vi "compressFiles.vi"(0 "show_bool_legal":bool=TRUE, 1 "original Path":path=path "S:/PNA_Data/L7KQF001-SD-R/SN-152440002_150901", 2 "重测原因":string, 3 "NetPathCompress2":path, 4 "EEPROMTF":bool=TRUE, 5 "Excel?":bool=TRUE, 6 "测试模式":string, 7 "db_VNA":string="L7KQF003-SD-R1;l7kqf003-sd-r1510090002;", 8 "P/N:":string, 9 "S/N:":string="152860001", 10 "测试线别":string, 12 "NetPathCompress1":path, 13 "NetCmdCompress":string, 14 "mis原始sn字符串":string, 15 "条码输出":string, 16 "eprm_datecode":string, 17 "eprm_dateAndsn":string, 20 "itsn_really":string, 21 "label_date":string, 23 "decimel_sn":string, 24 "label_sn":string, 25 "decimel_date":string, 27 "MO":string) -> ()   [LabVIEW 2011]
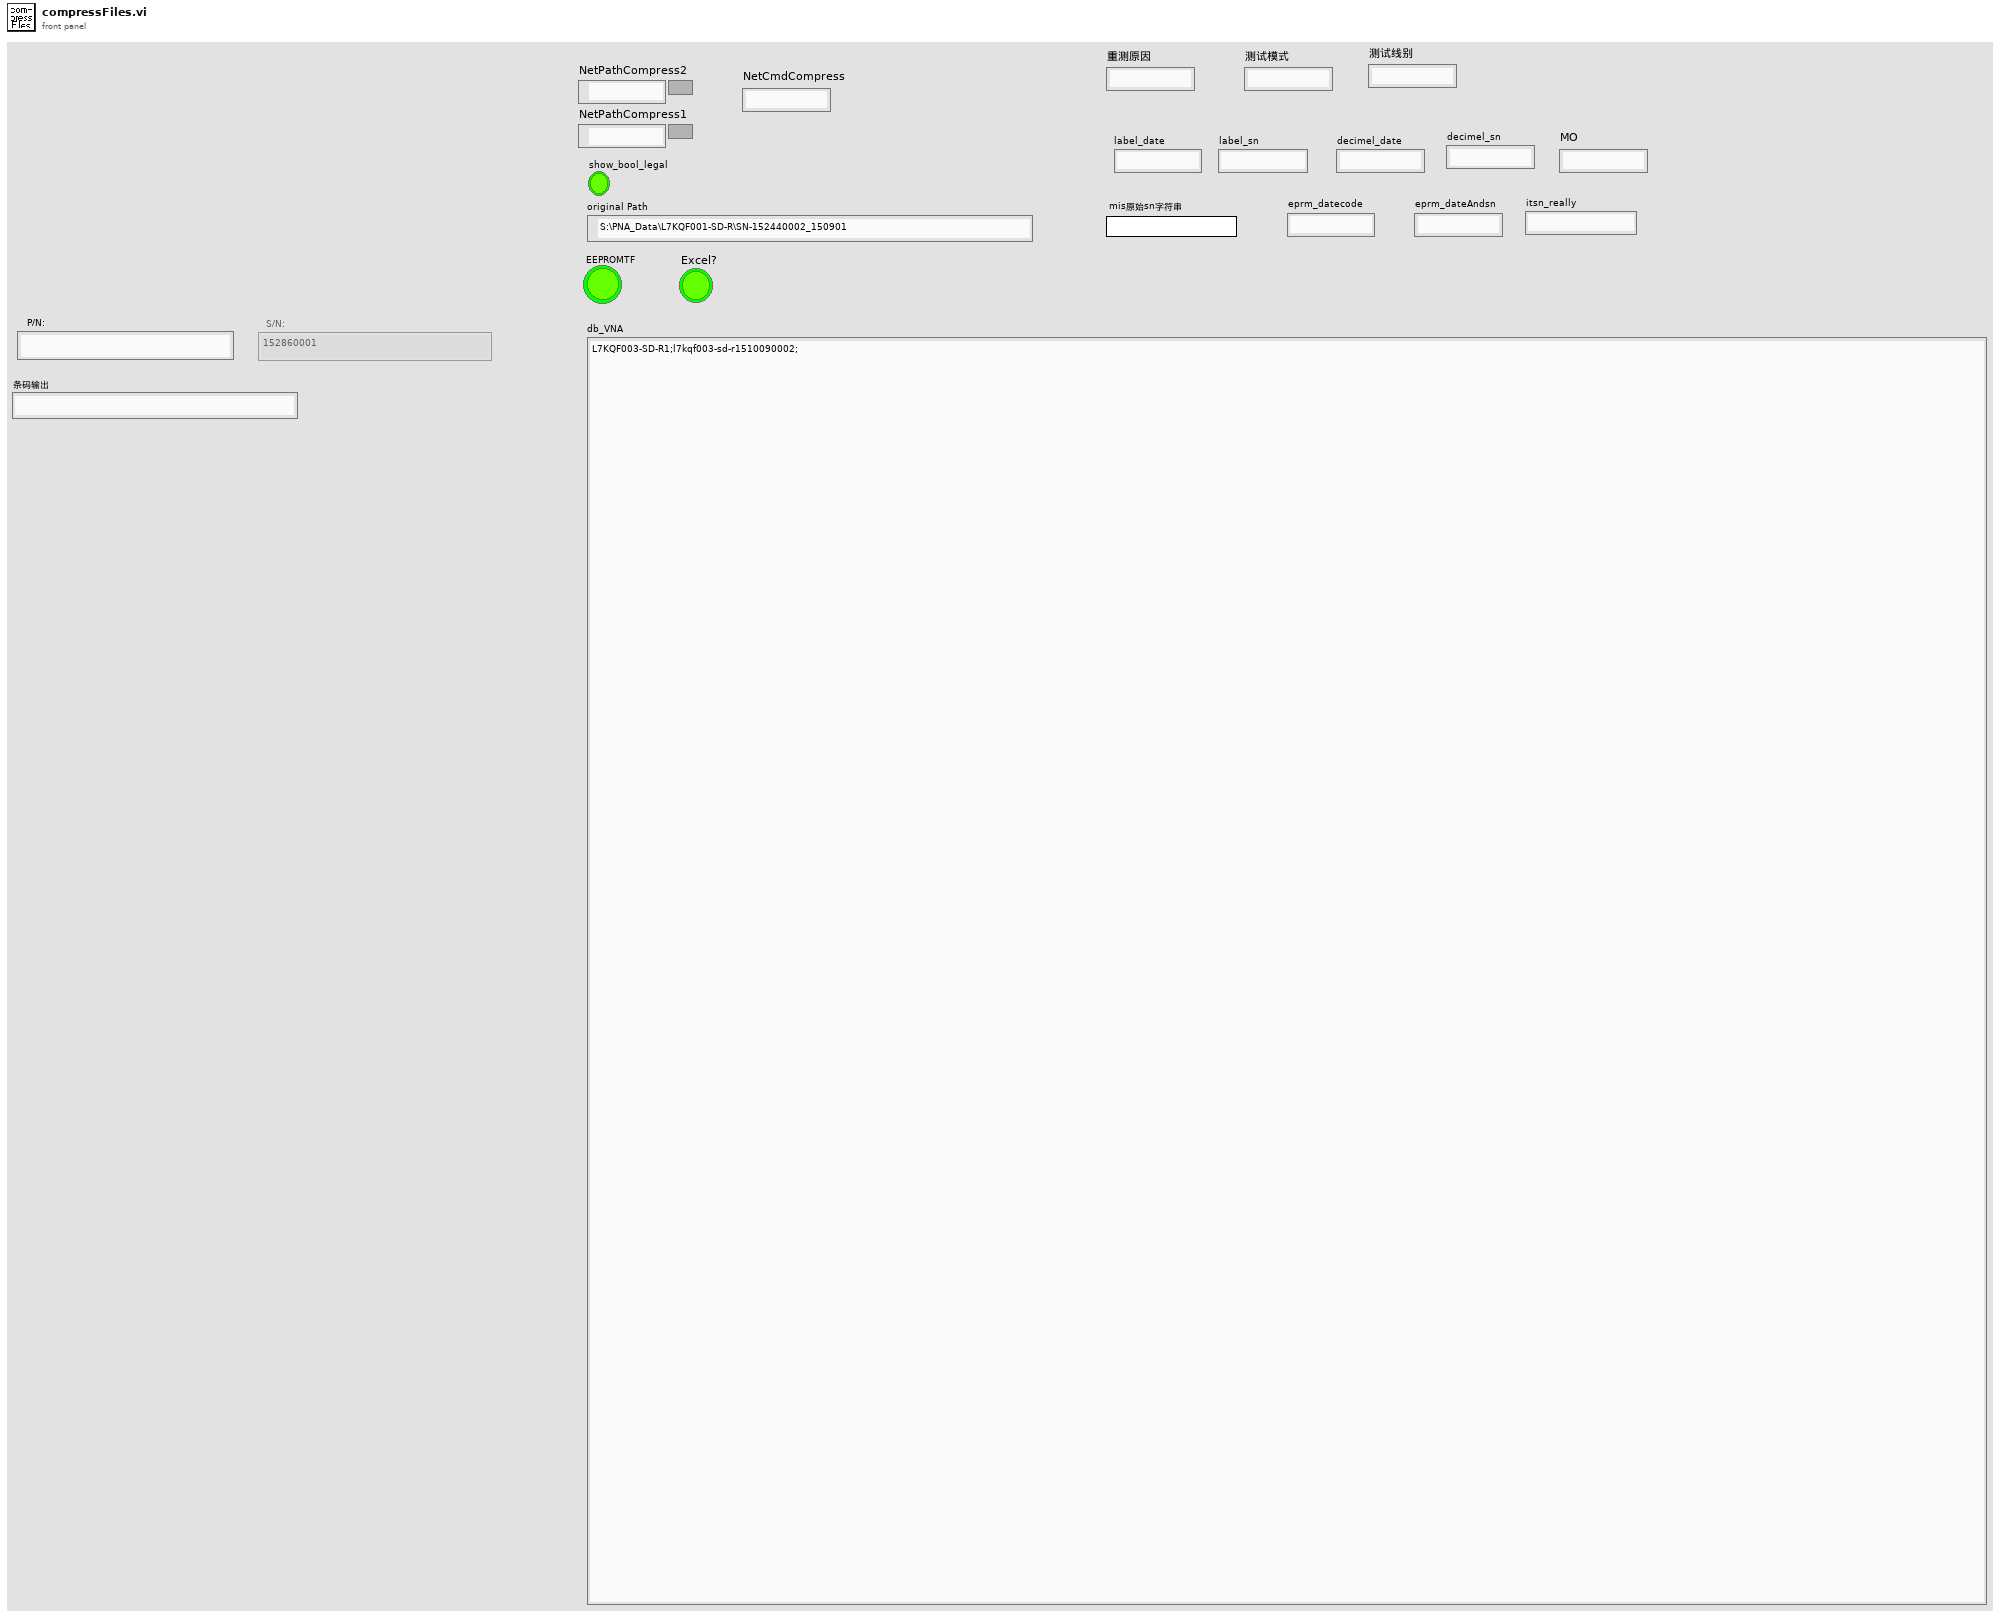
[diagram p1: front panel]
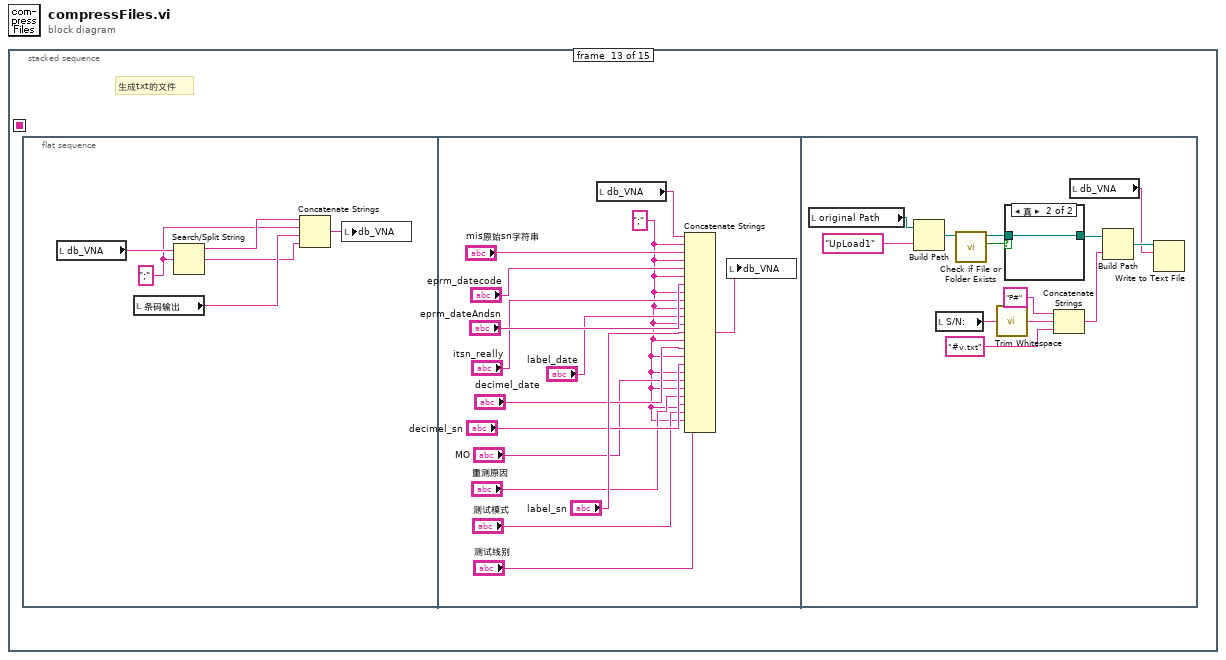
[diagram p0: block diagram]
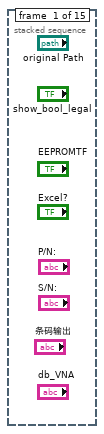
[diagram p2: hidden frame]
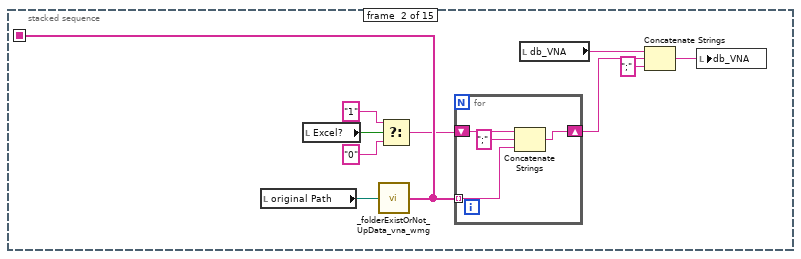
[diagram p3: hidden frame]
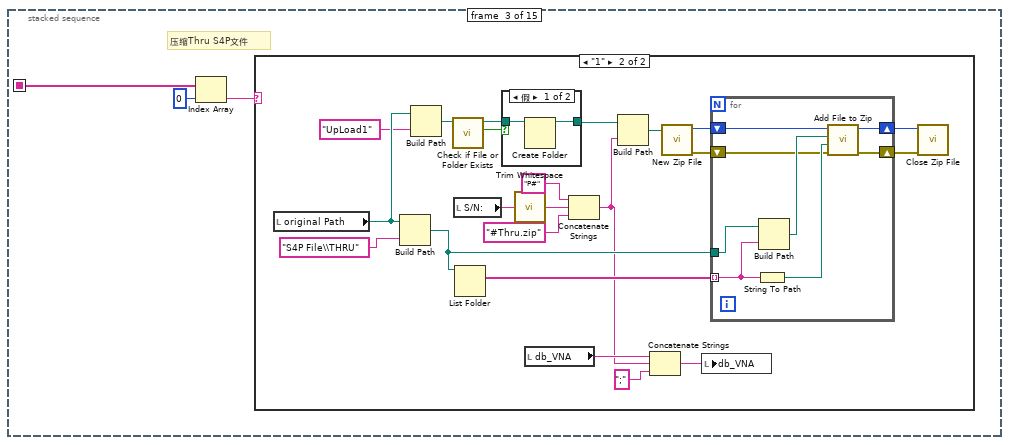
[diagram p4: hidden frame]
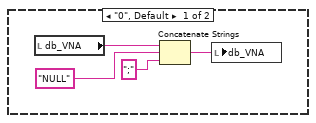
[diagram p5: hidden frame]
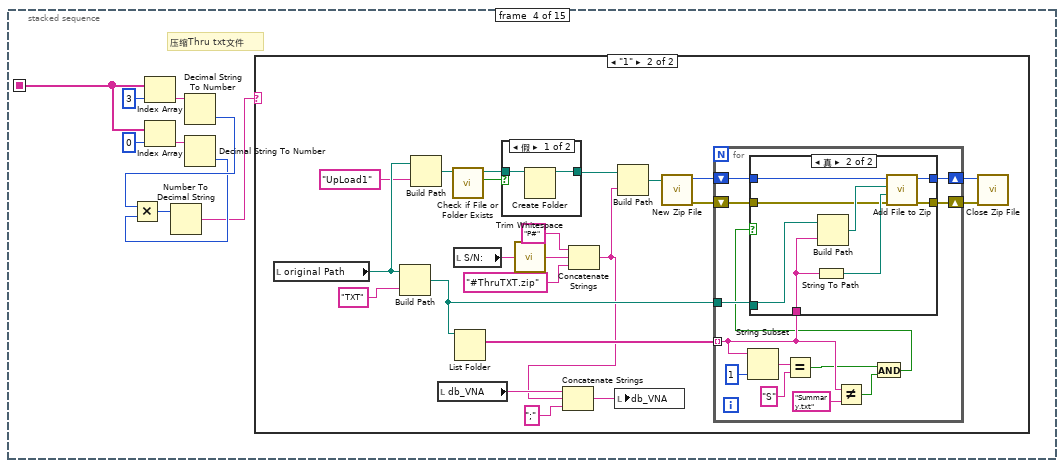
[diagram p7: hidden frame]
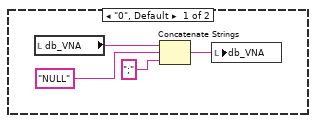
[diagram p8: hidden frame]
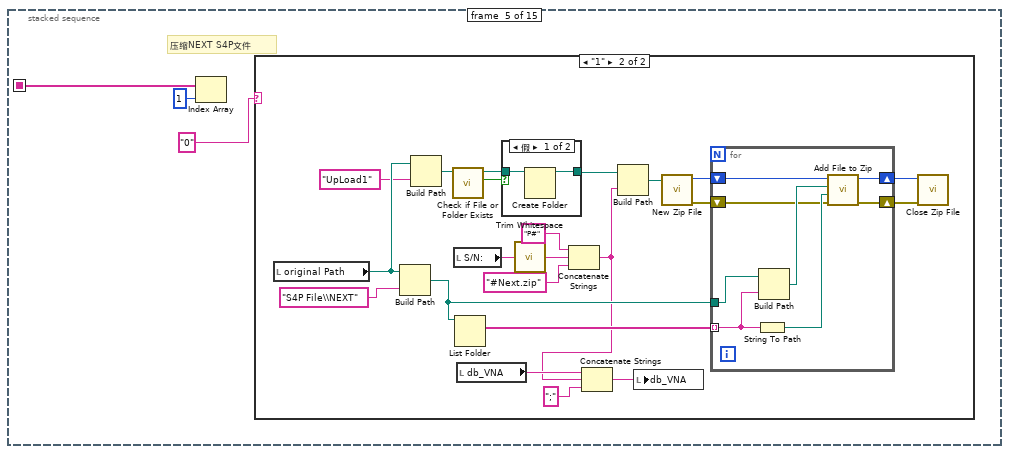
[diagram p11: hidden frame]
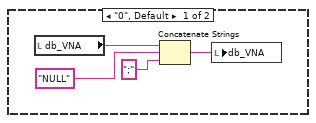
[diagram p12: hidden frame]
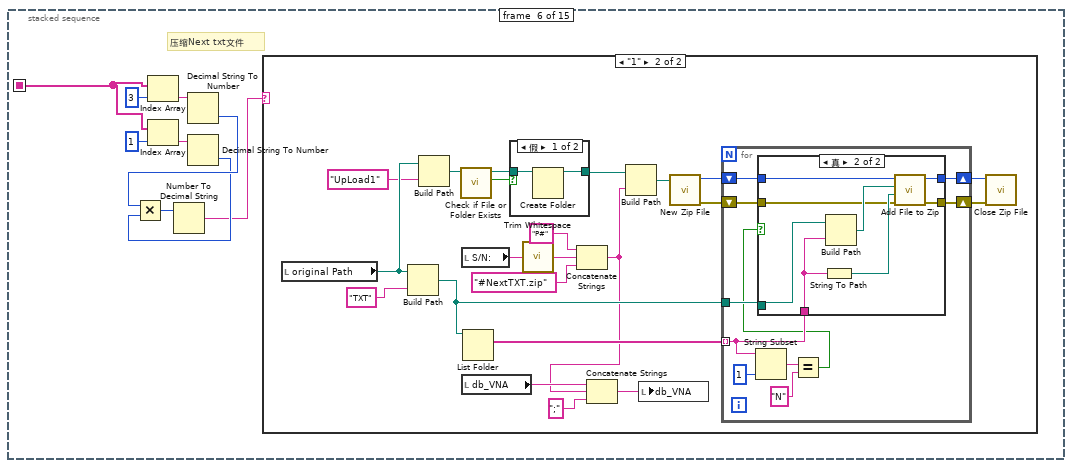
[diagram p14: hidden frame]
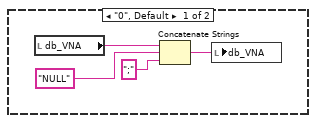
[diagram p15: hidden frame]
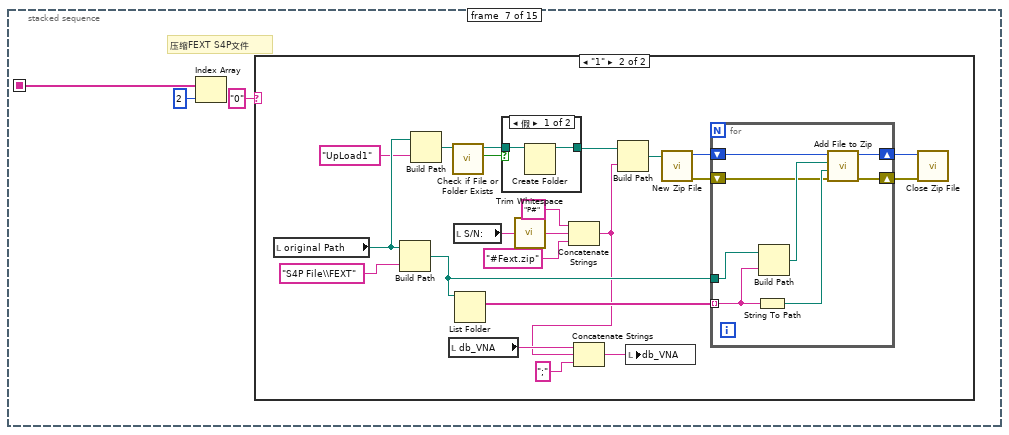
[diagram p18: hidden frame]
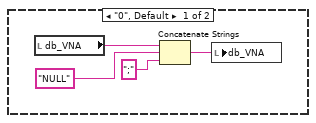
[diagram p19: hidden frame]
diagram:
  n1 = stacked-sequence {
    seq-local: [_ w2 _ _ _ _ _ _ _ _ _ _ _ _ _] -> [_ _ w17 w61 w118 w157 w216 w255 w314 w354 _ w458 _ _ _]
    frame #0 {
    }
    frame #1 {
      n2 = local read "original Path"() -> (w3:path)
      n3 = local read "Excel?"() -> (w10:bool)
      n4 = call "_folderExistOrNot_UpData_vna_wmg.vi"("基础路径"=w3) -> ("output"=w2:string[])
      n5 = Select(t="1", s=w10, f="0") -> (s? t:f=w1:string)
      n6 = for {
        tunnel: w2 -> [w12] mode=indexing
        shift-right: [w11] -> w5
        shift-left: w1 -> [w14]
        n7 = Concatenate Strings(w14, ";" ("字符串"), w12) -> (w11:string)
      }
      n8 = local read "db_VNA"() -> (w7:string)
      n9 = Concatenate Strings(w7, w5, ";" ("字符串")) -> (w6:string)
      n10 = local write "db_VNA"(w6) -> ()
    }
    frame #2 {
      # "压缩Thru S4P文件"
      n11 = Index Array(array=w17, index=0 ("索引")) -> (element=w15:string)
      n12 = case shown="\"1\"" w15 {
        frame "0", Default {
          n13 = local read "db_VNA"() -> (w21:string)
          n14 = Concatenate Strings(w21, "NULL", ";" ("字符串")) -> (w20:string)
          n15 = local write "db_VNA"(w20) -> ()
        }
        frame "1" {
          n16 = local read "original Path"() -> (w42:path)
          n17 = Build Path(base path=w42, name or relative path="S4P File\\THRU") -> (appended path=w31:path)
          n18 = Build Path(base path=w42, name or relative path="UpLoad1" ("名称或相对路径")) -> (appended path=w40:path)
          n19 = call <vilib>:"Check if File or Folder Exists.vi"("path"=w40) -> ("file or folder exists?"=w39:bool, "dup path"=w38:path)  [unwired: 8 in, 1 out]
          n20 = local read "S/N:"() -> (w37:string)
          n21 = List Folder(path=w31) -> (filenames=w32:string[])  [unwired: 3 in, 3 out]
          n22 = case shown="假" w39 {
            tunnel: w38 -> [w53 w54]
            tunnel: [w52 w54] -> w33
            frame False {
              n23 = Create Folder(path (use dialog)=w53) -> (created path=w52:path)  [unwired: 2 in, 2 out]
            }
            frame True {
            }
          }
          n24 = call <vilib>:"Trim Whitespace.vi"("string"=w37) -> ("trimmed string"=w36:string)  [unwired: 1 in]
          n25 = local read "db_VNA"() -> (w25:string)
          n26 = Concatenate Strings("P#", w36, "#Thru.zip") -> (w22:string)
          n27 = Build Path(base path=w33, name or relative path=w22) -> (appended path=w30:path)
          n28 = Concatenate Strings(w25, w22, ";" ("字符串")) -> (w24:string)
          n29 = call <vilib>:"New Zip File.vi"("target"=w30) -> ("error out"=w27:errorcluster, "zip file out"=w29:i64)  [unwired: 4 in, 1 out]
          n30 = local write "db_VNA"(w24) -> ()
          n31 = for {
            tunnel: w32 -> [w50] mode=indexing
            tunnel: w31 -> [w51]
            shift-right: [w48] -> w28
            shift-left: w29 -> [w49]
            shift-right: [w44] -> w26
            shift-left: w27 -> [w45]
            n32 = String To Path(string=w50) -> (path=w46:path)
            n33 = Build Path(base path=w51, name or relative path=w50) -> (appended path=w47:path)
            n34 = call <vilib>:"Add File to Zip.vi"("error in (no error)"=w45, "destination path in zip"=w46, "source file path"=w47, "zip file in"=w49) -> ("error out"=w44:errorcluster, "zip file out"=w48:i64)  [unwired: 6 in]
          }
          n35 = call <vilib>:"Close Zip File.vi"("error in (no error)"=w26, "zip file in"=w28) -> ()  [unwired: 5 in, 1 out]
        }
      }
    }
    frame #3 {
      # "压缩Thru txt文件"
      n36 = Index Array(array=w61, index=3 ("索引")) -> (element=w60:string)
      n37 = Index Array(array=w61, index=0 ("索引")) -> (element=w59:string)
      n38 = Decimal String To Number(string=w60) -> (number=w58:i32)  [unwired: 2 in, 1 out]
      n39 = Decimal String To Number(string=w59) -> (number=w57:i32)  [unwired: 2 in, 1 out]
      n40 = Multiply(x=w58, y=w57) -> (x*y=w56:i32)
      n41 = Number To Decimal String(number=w56) -> (decimal integer string=w55:string)  [unwired: 1 in]
      n42 = case shown="\"1\"" w55 {
        frame "0", Default {
          n43 = local read "db_VNA"() -> (w67:string)
          n44 = Concatenate Strings(w67, "NULL", ";" ("字符串")) -> (w66:string)
          n45 = local write "db_VNA"(w66) -> ()
        }
        frame "1" {
          n46 = local read "original Path"() -> (w88:path)
          n47 = Build Path(base path=w88, name or relative path="TXT") -> (appended path=w77:path)
          n48 = Build Path(base path=w88, name or relative path="UpLoad1" ("名称或相对路径")) -> (appended path=w86:path)
          n49 = local read "db_VNA"() -> (w71:string)
          n50 = call <vilib>:"Check if File or Folder Exists.vi"("path"=w86) -> ("file or folder exists?"=w85:bool, "dup path"=w84:path)  [unwired: 8 in, 1 out]
          n51 = local read "S/N:"() -> (w83:string)
          n52 = List Folder(path=w77) -> (filenames=w78:string[])  [unwired: 3 in, 3 out]
          n53 = case shown="假" w85 {
            tunnel: w84 -> [w114 w115]
            tunnel: [w113 w115] -> w79
            frame False {
              n54 = Create Folder(path (use dialog)=w114) -> (created path=w113:path)  [unwired: 2 in, 2 out]
            }
            frame True {
            }
          }
          n55 = call <vilib>:"Trim Whitespace.vi"("string"=w83) -> ("trimmed string"=w82:string)  [unwired: 1 in]
          n56 = Concatenate Strings("P#", w82, "#ThruTXT.zip") -> (w68:string)
          n57 = Concatenate Strings(w71, w68, ";" ("字符串")) -> (w70:string)
          n58 = local write "db_VNA"(w70) -> ()
          n59 = Build Path(base path=w79, name or relative path=w68) -> (appended path=w76:path)
          n60 = call <vilib>:"New Zip File.vi"("target"=w76) -> ("error out"=w73:errorcluster, "zip file out"=w75:i64)  [unwired: 4 in, 1 out]
          n61 = for {
            tunnel: w78 -> [w94] mode=indexing
            tunnel: w77 -> [w102]
            shift-right: [w100] -> w74
            shift-left: w75 -> [w101]
            shift-right: [w98] -> w72
            shift-left: w73 -> [w99]
            n62 = String Subset(string=w94, length (rest)=1 ("长度（剩余）")) -> (substring=w96:string)  [unwired: 1 in]
            n63 = Equal?(x=w96, y="S") -> (x = y?=w91:bool)
            n64 = Not Equal?(x=w94, y="Summary.txt") -> (x != y?=w92:bool)
            n65 = And(x=w91, y=w92) -> (x .and. y?=w90:bool)
            n66 = case shown="真" w90 {
              tunnel: w102 -> [_ w112]
              tunnel: w101 -> [w104 w111]
              tunnel: [w104 w110] -> w100
              tunnel: w99 -> [w103 w107]
              tunnel: [w103 w106] -> w98
              tunnel: w94 -> [_ w105]
              frame False {
              }
              frame True {
                n67 = String To Path(string=w105) -> (path=w108:path)
                n68 = Build Path(base path=w112, name or relative path=w105) -> (appended path=w109:path)
                n69 = call <vilib>:"Add File to Zip.vi"("error in (no error)"=w107, "destination path in zip"=w108, "source file path"=w109, "zip file in"=w111) -> ("error out"=w106:errorcluster, "zip file out"=w110:i64)  [unwired: 6 in]
              }
            }
          }
          n70 = call <vilib>:"Close Zip File.vi"("error in (no error)"=w72, "zip file in"=w74) -> ()  [unwired: 5 in, 1 out]
        }
      }
    }
    frame #4 {
      # "压缩NEXT S4P文件"
      n71 = Index Array(array=w118, index=1 ("索引")) -> ()  [unwired: 1 out]
      n72 = case shown="\"1\"" "0" {
        frame "0", Default {
          n73 = local read "db_VNA"() -> (w122:string)
          n74 = Concatenate Strings(w122, "NULL", ";" ("字符串")) -> (w121:string)
          n75 = local write "db_VNA"(w121) -> ()
        }
        frame "1" {
          n76 = local read "original Path"() -> (w143:path)
          n77 = Build Path(base path=w143, name or relative path="S4P File\\NEXT") -> (appended path=w132:path)
          n78 = Build Path(base path=w143, name or relative path="UpLoad1" ("名称或相对路径")) -> (appended path=w141:path)
          n79 = call <vilib>:"Check if File or Folder Exists.vi"("path"=w141) -> ("file or folder exists?"=w140:bool, "dup path"=w139:path)  [unwired: 8 in, 1 out]
          n80 = local read "S/N:"() -> (w138:string)
          n81 = List Folder(path=w132) -> (filenames=w133:string[])  [unwired: 3 in, 3 out]
          n82 = local read "db_VNA"() -> (w124:string)
          n83 = case shown="假" w140 {
            tunnel: w139 -> [w154 w155]
            tunnel: [w153 w155] -> w134
            frame False {
              n84 = Create Folder(path (use dialog)=w154) -> (created path=w153:path)  [unwired: 2 in, 2 out]
            }
            frame True {
            }
          }
          n85 = call <vilib>:"Trim Whitespace.vi"("string"=w138) -> ("trimmed string"=w137:string)  [unwired: 1 in]
          n86 = Concatenate Strings("P#", w137, "#Next.zip") -> (w123:string)
          n87 = Concatenate Strings(w124, w123, ";" ("字符串")) -> (w125:string)
          n88 = Build Path(base path=w134, name or relative path=w123) -> (appended path=w131:path)
          n89 = local write "db_VNA"(w125) -> ()
          n90 = call <vilib>:"New Zip File.vi"("target"=w131) -> ("error out"=w128:errorcluster, "zip file out"=w130:i64)  [unwired: 4 in, 1 out]
          n91 = for {
            tunnel: w133 -> [w151] mode=indexing
            tunnel: w132 -> [w152]
            shift-right: [w149] -> w129
            shift-left: w130 -> [w150]
            shift-right: [w145] -> w127
            shift-left: w128 -> [w146]
            n92 = String To Path(string=w151) -> (path=w147:path)
            n93 = Build Path(base path=w152, name or relative path=w151) -> (appended path=w148:path)
            n94 = call <vilib>:"Add File to Zip.vi"("error in (no error)"=w146, "destination path in zip"=w147, "source file path"=w148, "zip file in"=w150) -> ("error out"=w145:errorcluster, "zip file out"=w149:i64)  [unwired: 6 in]
          }
          n95 = call <vilib>:"Close Zip File.vi"("error in (no error)"=w127, "zip file in"=w129) -> ()  [unwired: 5 in, 1 out]
        }
      }
    }
    frame #5 {
      # "压缩Next txt文件"
      n96 = Index Array(array=w157, index=3 ("索引")) -> (element=w162:string)
      n97 = Index Array(array=w157, index=1 ("索引")) -> (element=w161:string)
      n98 = Decimal String To Number(string=w162) -> (number=w160:i32)  [unwired: 2 in, 1 out]
      n99 = Decimal String To Number(string=w161) -> (number=w159:i32)  [unwired: 2 in, 1 out]
      n100 = Multiply(x=w160, y=w159) -> (x*y=w158:i32)
      n101 = Number To Decimal String(number=w158) -> (decimal integer string=w156:string)  [unwired: 1 in]
      n102 = case shown="\"1\"" w156 {
        frame "0", Default {
          n103 = local read "db_VNA"() -> (w168:string)
          n104 = Concatenate Strings(w168, "NULL", ";" ("字符串")) -> (w167:string)
          n105 = local write "db_VNA"(w167) -> ()
        }
        frame "1" {
          n106 = local read "original Path"() -> (w189:path)
          n107 = Build Path(base path=w189, name or relative path="TXT") -> (appended path=w178:path)
          n108 = Build Path(base path=w189, name or relative path="UpLoad1" ("名称或相对路径")) -> (appended path=w187:path)
          n109 = call <vilib>:"Check if File or Folder Exists.vi"("path"=w187) -> ("file or folder exists?"=w186:bool, "dup path"=w185:path)  [unwired: 8 in, 1 out]
          n110 = local read "S/N:"() -> (w184:string)
          n111 = local read "db_VNA"() -> (w172:string)
          n112 = List Folder(path=w178) -> (filenames=w179:string[])  [unwired: 3 in, 3 out]
          n113 = case shown="假" w186 {
            tunnel: w185 -> [w212 w213]
            tunnel: [w211 w213] -> w180
            frame False {
              n114 = Create Folder(path (use dialog)=w212) -> (created path=w211:path)  [unwired: 2 in, 2 out]
            }
            frame True {
            }
          }
          n115 = call <vilib>:"Trim Whitespace.vi"("string"=w184) -> ("trimmed string"=w183:string)  [unwired: 1 in]
          n116 = Concatenate Strings("P#", w183, "#NextTXT.zip") -> (w169:string)
          n117 = Concatenate Strings(w172, w169, ";" ("字符串")) -> (w171:string)
          n118 = Build Path(base path=w180, name or relative path=w169) -> (appended path=w177:path)
          n119 = local write "db_VNA"(w171) -> ()
          n120 = call <vilib>:"New Zip File.vi"("target"=w177) -> ("error out"=w174:errorcluster, "zip file out"=w176:i64)  [unwired: 4 in, 1 out]
          n121 = for {
            tunnel: w179 -> [w195] mode=indexing
            tunnel: w178 -> [w200]
            shift-right: [w198] -> w175
            shift-left: w176 -> [w199]
            shift-right: [w196] -> w173
            shift-left: w174 -> [w197]
            n122 = String Subset(string=w195, length (rest)=1 ("长度（剩余）")) -> (substring=w193:string)  [unwired: 1 in]
            n123 = Equal?(x=w193, y="N") -> (x = y?=w191:bool)
            n124 = case shown="真" w191 {
              tunnel: w200 -> [_ w210]
              tunnel: w199 -> [w202 w209]
              tunnel: [w202 w208] -> w198
              tunnel: w197 -> [w201 w205]
              tunnel: [w201 w204] -> w196
              tunnel: w195 -> [_ w203]
              frame False {
              }
              frame True {
                n125 = String To Path(string=w203) -> (path=w206:path)
                n126 = Build Path(base path=w210, name or relative path=w203) -> (appended path=w207:path)
                n127 = call <vilib>:"Add File to Zip.vi"("error in (no error)"=w205, "destination path in zip"=w206, "source file path"=w207, "zip file in"=w209) -> ("error out"=w204:errorcluster, "zip file out"=w208:i64)  [unwired: 6 in]
              }
            }
          }
          n128 = call <vilib>:"Close Zip File.vi"("error in (no error)"=w173, "zip file in"=w175) -> ()  [unwired: 5 in, 1 out]
        }
      }
    }
    frame #6 {
      # "压缩FEXT S4P文件"
      n129 = Index Array(array=w216, index=2 ("索引")) -> ()  [unwired: 1 out]
      n130 = case shown="\"1\"" "0" {
        frame "0", Default {
          n131 = local read "db_VNA"() -> (w220:string)
          n132 = Concatenate Strings(w220, "NULL", ";" ("字符串")) -> (w219:string)
          n133 = local write "db_VNA"(w219) -> ()
        }
        frame "1" {
          n134 = local read "original Path"() -> (w241:path)
          n135 = Build Path(base path=w241, name or relative path="S4P File\\FEXT") -> (appended path=w230:path)
          n136 = Build Path(base path=w241, name or relative path="UpLoad1" ("名称或相对路径")) -> (appended path=w239:path)
          n137 = local read "db_VNA"() -> (w222:string)
          n138 = call <vilib>:"Check if File or Folder Exists.vi"("path"=w239) -> ("file or folder exists?"=w238:bool, "dup path"=w237:path)  [unwired: 8 in, 1 out]
          n139 = local read "S/N:"() -> (w236:string)
          n140 = List Folder(path=w230) -> (filenames=w231:string[])  [unwired: 3 in, 3 out]
          n141 = case shown="假" w238 {
            tunnel: w237 -> [w252 w253]
            tunnel: [w251 w253] -> w232
            frame False {
              n142 = Create Folder(path (use dialog)=w252) -> (created path=w251:path)  [unwired: 2 in, 2 out]
            }
            frame True {
            }
          }
          n143 = call <vilib>:"Trim Whitespace.vi"("string"=w236) -> ("trimmed string"=w235:string)  [unwired: 1 in]
          n144 = Concatenate Strings("P#", w235, "#Fext.zip") -> (w221:string)
          n145 = Concatenate Strings(w222, w221, ";" ("字符串")) -> (w223:string)
          n146 = Build Path(base path=w232, name or relative path=w221) -> (appended path=w229:path)
          n147 = local write "db_VNA"(w223) -> ()
          n148 = call <vilib>:"New Zip File.vi"("target"=w229) -> ("error out"=w226:errorcluster, "zip file out"=w228:i64)  [unwired: 4 in, 1 out]
          n149 = for {
            tunnel: w231 -> [w249] mode=indexing
            tunnel: w230 -> [w250]
            shift-right: [w247] -> w227
            shift-left: w228 -> [w248]
            shift-right: [w243] -> w225
            shift-left: w226 -> [w244]
            n150 = String To Path(string=w249) -> (path=w245:path)
            n151 = Build Path(base path=w250, name or relative path=w249) -> (appended path=w246:path)
            n152 = call <vilib>:"Add File to Zip.vi"("error in (no error)"=w244, "destination path in zip"=w245, "source file path"=w246, "zip file in"=w248) -> ("error out"=w243:errorcluster, "zip file out"=w247:i64)  [unwired: 6 in]
          }
          n153 = call <vilib>:"Close Zip File.vi"("error in (no error)"=w225, "zip file in"=w227) -> ()  [unwired: 5 in, 1 out]
        }
      }
    }
    frame #7 {
      # "压缩Fext txt文件"
      n154 = Index Array(array=w255, index=3 ("索引")) -> (element=w260:string)
      n155 = Index Array(array=w255, index=2 ("索引")) -> (element=w259:string)
      n156 = Decimal String To Number(string=w260) -> (number=w258:i32)  [unwired: 2 in, 1 out]
      n157 = Decimal String To Number(string=w259) -> (number=w257:i32)  [unwired: 2 in, 1 out]
      n158 = Multiply(x=w258, y=w257) -> (x*y=w256:i32)
      n159 = Number To Decimal String(number=w256) -> (decimal integer string=w254:string)  [unwired: 1 in]
      n160 = case shown="\"1\"" w254 {
        frame "0", Default {
          n161 = local read "db_VNA"() -> (w266:string)
          n162 = Concatenate Strings(w266, "NULL", ";" ("字符串")) -> (w265:string)
          n163 = local write "db_VNA"(w265) -> ()
        }
        frame "1" {
          n164 = local read "original Path"() -> (w287:path)
          n165 = Build Path(base path=w287, name or relative path="TXT") -> (appended path=w276:path)
          n166 = Build Path(base path=w287, name or relative path="UpLoad1" ("名称或相对路径")) -> (appended path=w285:path)
          n167 = local read "db_VNA"() -> (w270:string)
          n168 = call <vilib>:"Check if File or Folder Exists.vi"("path"=w285) -> ("file or folder exists?"=w284:bool, "dup path"=w283:path)  [unwired: 8 in, 1 out]
          n169 = local read "S/N:"() -> (w282:string)
          n170 = List Folder(path=w276) -> (filenames=w277:string[])  [unwired: 3 in, 3 out]
          n171 = case shown="假" w284 {
            tunnel: w283 -> [w310 w311]
            tunnel: [w309 w311] -> w278
            frame False {
              n172 = Create Folder(path (use dialog)=w310) -> (created path=w309:path)  [unwired: 2 in, 2 out]
            }
            frame True {
            }
          }
          n173 = call <vilib>:"Trim Whitespace.vi"("string"=w282) -> ("trimmed string"=w281:string)  [unwired: 1 in]
          n174 = Concatenate Strings("P#", w281, "#FextTXT.zip") -> (w267:string)
          n175 = Concatenate Strings(w270, w267, ";" ("字符串")) -> (w269:string)
          n176 = Build Path(base path=w278, name or relative path=w267) -> (appended path=w275:path)
          n177 = local write "db_VNA"(w269) -> ()
          n178 = call <vilib>:"New Zip File.vi"("target"=w275) -> ("error out"=w272:errorcluster, "zip file out"=w274:i64)  [unwired: 4 in, 1 out]
          n179 = for {
            tunnel: w277 -> [w293] mode=indexing
            tunnel: w276 -> [w298]
            shift-right: [w296] -> w273
            shift-left: w274 -> [w297]
            shift-right: [w294] -> w271
            shift-left: w272 -> [w295]
            n180 = String Subset(string=w293, length (rest)=1 ("长度（剩余）")) -> (substring=w291:string)  [unwired: 1 in]
            n181 = Equal?(x=w291, y="F") -> (x = y?=w289:bool)
            n182 = case shown="真" w289 {
              tunnel: w298 -> [_ w308]
              tunnel: w297 -> [w300 w307]
              tunnel: [w300 w306] -> w296
              tunnel: w295 -> [w299 w303]
              tunnel: [w299 w302] -> w294
              tunnel: w293 -> [_ w301]
              frame False {
              }
              frame True {
                n183 = String To Path(string=w301) -> (path=w304:path)
                n184 = Build Path(base path=w308, name or relative path=w301) -> (appended path=w305:path)
                n185 = call <vilib>:"Add File to Zip.vi"("error in (no error)"=w303, "destination path in zip"=w304, "source file path"=w305, "zip file in"=w307) -> ("error out"=w302:errorcluster, "zip file out"=w306:i64)  [unwired: 6 in]
              }
            }
          }
          n186 = call <vilib>:"Close Zip File.vi"("error in (no error)"=w271, "zip file in"=w273) -> ()  [unwired: 5 in, 1 out]
        }
      }
    }
    frame #8 {
      # "压缩全部TXT文件，20170214 Figoba"
      # "压缩其他 txt文件"
      n187 = Index Array(array=w314, index=3 ("索引")) -> (element=w312:string)
      n188 = case shown="\"1\"" w312 {
        frame "0", Default {
          n189 = local read "db_VNA"() -> (w318:string)
          n190 = Concatenate Strings(w318, "NULL", ";" ("字符串")) -> (w317:string)
          n191 = local write "db_VNA"(w317) -> ()
        }
        frame "1" {
          n192 = local read "original Path"() -> (w325:path)
          n193 = Build Path(base path=w325, name or relative path="TXT" ("名称或相对路径")) -> (appended path=w324:path)
          n194 = Build Path(base path=w325, name or relative path="UpLoad1" ("名称或相对路径")) -> (appended path=w339:path)
          n195 = local read "db_VNA"() -> (w322:string)
          n196 = call <vilib>:"Check if File or Folder Exists.vi"("path"=w339) -> ("file or folder exists?"=w338:bool, "dup path"=w337:path)  [unwired: 8 in, 1 out]
          n197 = local read "S/N:"() -> (w336:string)
          n198 = List Folder(path=w324) -> (filenames=w331:string[])  [unwired: 3 in, 3 out]
          n199 = case shown="假" w338 {
            tunnel: w337 -> [w350 w351]
            tunnel: [w349 w351] -> w332
            frame False {
              n200 = Create Folder(path (use dialog)=w350) -> (created path=w349:path)  [unwired: 2 in, 2 out]
            }
            frame True {
            }
          }
          n201 = call <vilib>:"Trim Whitespace.vi"("string"=w336) -> ("trimmed string"=w335:string)  [unwired: 1 in]
          n202 = Concatenate Strings("P#", w335, "#TXT.zip") -> (w319:string)
          n203 = Concatenate Strings(w322, w319, ";" ("字符串")) -> (w321:string)
          n204 = local write "db_VNA"(w321) -> ()
          n205 = Build Path(base path=w332, name or relative path=w319) -> (appended path=w330:path)
          n206 = call <vilib>:"New Zip File.vi"("target"=w330) -> ("error out"=w327:errorcluster, "zip file out"=w329:i64)  [unwired: 4 in, 1 out]
          n207 = for {
            tunnel: w331 -> [w341] mode=indexing
            tunnel: w324 -> [w348]
            shift-right: [w346] -> w328
            shift-left: w329 -> [w347]
            shift-right: [w344] -> w326
            shift-left: w327 -> [w345]
            n208 = String To Path(string=w341) -> (path=w342:path)
            n209 = Build Path(base path=w348, name or relative path=w341) -> (appended path=w343:path)
            n210 = call <vilib>:"Add File to Zip.vi"("error in (no error)"=w345, "destination path in zip"=w342, "source file path"=w343, "zip file in"=w347) -> ("error out"=w344:errorcluster, "zip file out"=w346:i64)  [unwired: 6 in]
          }
          n211 = call <vilib>:"Close Zip File.vi"("error in (no error)"=w326, "zip file in"=w328) -> ()  [unwired: 5 in, 1 out]
        }
      }
    }
    frame #9 {
      # "压缩PDF文件"
      n212 = Index Array(array=w354, index=5 ("索引")) -> (element=w352:string)
      n213 = case shown="\"1\"" w352 {
        frame "0", Default {
          n214 = local read "db_VNA"() -> (w358:string)
          n215 = Concatenate Strings(w358, "NULL", ";" ("字符串")) -> (w357:string)
          n216 = local write "db_VNA"(w357) -> ()
        }
        frame "1" {
          n217 = local read "original Path"() -> (w363:path)
          n218 = Build Path(base path=w363, name or relative path="UpLoad1" ("名称或相对路径")) -> (appended path=w377:path)
          n219 = local read "db_VNA"() -> (w362:string)
          n220 = call <vilib>:"Check if File or Folder Exists.vi"("path"=w377) -> ("file or folder exists?"=w376:bool, "dup path"=w375:path)  [unwired: 8 in, 1 out]
          n221 = local read "S/N:"() -> (w374:string)
          n222 = List Folder(path=w363) -> (filenames=w369:string[])  [unwired: 3 in, 3 out]
          n223 = case shown="假" w376 {
            tunnel: w375 -> [w403 w404]
            tunnel: [w402 w404] -> w370
            frame False {
              n224 = Create Folder(path (use dialog)=w403) -> (created path=w402:path)  [unwired: 2 in, 2 out]
            }
            frame True {
            }
          }
          n225 = call <vilib>:"Trim Whitespace.vi"("string"=w374) -> ("trimmed string"=w373:string)  [unwired: 1 in]
          n226 = Concatenate Strings("P#", w373, "#PDF.zip") -> (w359:string)
          n227 = Concatenate Strings(w362, w359, ";" ("字符串")) -> (w361:string)
          n228 = Build Path(base path=w370, name or relative path=w359) -> (appended path=w368:path)
          n229 = local write "db_VNA"(w361) -> ()
          n230 = call <vilib>:"New Zip File.vi"("target"=w368) -> ("error out"=w365:errorcluster, "zip file out"=w367:i64)  [unwired: 4 in, 1 out]
          n231 = for {
            tunnel: w369 -> [w384] mode=indexing
            tunnel: w363 -> [w391]
            shift-right: [w389] -> w366
            shift-left: w367 -> [w390]
            shift-right: [w387] -> w364
            shift-left: w365 -> [w388]
            n232 = Search and Replace String(input string=w384, search string=".xls" ("搜索字符串")) -> (number of replacements=w383:i32)  [unwired: 6 in, 3 out]
            n233 = Search and Replace String(input string=w384, search string=".xlsx" ("搜索字符串")) -> (number of replacements=w382:i32)  [unwired: 6 in, 3 out]
            n234 = Greater Than 0?(x=w383) -> (x > 0?=w381:bool)
            n235 = Greater Than 0?(x=w382) -> (x > 0?=w380:bool)
            n236 = Or(x=w381, y=w380) -> (x .or. y?=w379:bool)
            n237 = case shown="真" w379 {
              tunnel: w391 -> [_ w401]
              tunnel: w390 -> [w393 w400]
              tunnel: [w393 w399] -> w389
              tunnel: w388 -> [w392 w396]
              tunnel: [w392 w395] -> w387
              tunnel: w384 -> [_ w394]
              frame False {
              }
              frame True {
                n238 = String To Path(string=w394) -> (path=w397:path)
                n239 = Build Path(base path=w401, name or relative path=w394) -> (appended path=w398:path)
                n240 = call <vilib>:"Add File to Zip.vi"("error in (no error)"=w396, "destination path in zip"=w397, "source file path"=w398, "zip file in"=w400) -> ("error out"=w395:errorcluster, "zip file out"=w399:i64)  [unwired: 6 in]
              }
            }
          }
          n241 = call <vilib>:"Close Zip File.vi"("error in (no error)"=w364, "zip file in"=w366) -> ()  [unwired: 5 in, 1 out]
        }
      }
    }
    frame #10 {
      # "压缩EEPROM文件"
      n242 = local read "EEPROMTF"() -> (w407:bool)
      n243 = local read "show_bool_legal"() -> (w405:bool)
      n244 = And(x=w407, y=w405) -> (x .and. y?=w406:bool)
      n245 = case shown="假" w406 {
        frame False {
          n246 = local read "db_VNA"() -> (w411:string)
          n247 = Concatenate Strings(w411, "NULL", ";" ("字符串")) -> (w410:string)
          n248 = local write "db_VNA"(w410) -> ()
        }
        frame True {
          n249 = local read "original Path"() -> (w414:path)
          n250 = Build Path(base path=w414, name or relative path="TXT" ("名称或相对路径")) -> (appended path=w413:path)
          n251 = Build Path(base path=w414, name or relative path="UpLoad1" ("名称或相对路径")) -> (appended path=w432:path)
          n252 = local read "db_VNA"() -> (w418:string)
          n253 = call <vilib>:"Check if File or Folder Exists.vi"("path"=w432) -> ("file or folder exists?"=w431:bool, "dup path"=w430:path)  [unwired: 8 in, 1 out]
          n254 = local read "S/N:"() -> (w429:string)
          n255 = List Folder(path=w413) -> (filenames=w424:string[])  [unwired: 3 in, 3 out]
          n256 = case shown="假" w431 {
            tunnel: w430 -> [w454 w455]
            tunnel: [w453 w455] -> w425
            frame False {
              n257 = Create Folder(path (use dialog)=w454) -> (created path=w453:path)  [unwired: 2 in, 2 out]
            }
            frame True {
            }
          }
          n258 = call <vilib>:"Trim Whitespace.vi"("string"=w429) -> ("trimmed string"=w428:string)  [unwired: 1 in]
          n259 = Concatenate Strings("P#", w428, "#EEPROM.zip") -> (w415:string)
          n260 = Concatenate Strings(w418, w415, ";" ("字符串")) -> (w417:string)
          n261 = local write "db_VNA"(w417) -> ()
          n262 = Build Path(base path=w425, name or relative path=w415) -> (appended path=w423:path)
          n263 = call <vilib>:"New Zip File.vi"("target"=w423) -> ("error out"=w420:errorcluster, "zip file out"=w422:i64)  [unwired: 4 in, 1 out]
          n264 = for {
            tunnel: w424 -> [w436] mode=indexing
            tunnel: w413 -> [w442]
            shift-right: [w440] -> w421
            shift-left: w422 -> [w441]
            shift-right: [w438] -> w419
            shift-left: w420 -> [w439]
            n265 = Search and Replace String(input string=w436, search string="EEPROM" ("搜索字符串")) -> (number of replacements=w435:i32)  [unwired: 6 in, 3 out]
            n266 = Greater Than 0?(x=w435) -> (x > 0?=w434:bool)
            n267 = case shown="真" w434 {
              tunnel: w442 -> [_ w452]
              tunnel: w441 -> [w444 w451]
              tunnel: [w444 w450] -> w440
              tunnel: w439 -> [w443 w447]
              tunnel: [w443 w446] -> w438
              tunnel: w436 -> [_ w445]
              frame False {
              }
              frame True {
                n268 = String To Path(string=w445) -> (path=w448:path)
                n269 = Build Path(base path=w452, name or relative path=w445) -> (appended path=w449:path)
                n270 = call <vilib>:"Add File to Zip.vi"("error in (no error)"=w447, "destination path in zip"=w448, "source file path"=w449, "zip file in"=w451) -> ("error out"=w446:errorcluster, "zip file out"=w450:i64)  [unwired: 6 in]
              }
            }
          }
          n271 = call <vilib>:"Close Zip File.vi"("error in (no error)"=w419, "zip file in"=w421) -> ()  [unwired: 5 in, 1 out]
        }
      }
    }
    frame #11 {
      # "压缩Suammary 文件"
      n272 = Index Array(array=w458, index=3 ("索引")) -> (element=w456:string)
      n273 = case shown="\"1\"" w456 {
        frame "0", Default {
          n274 = local read "db_VNA"() -> (w462:string)
          n275 = Concatenate Strings(w462, "NULL", ";" ("字符串")) -> (w461:string)
          n276 = local write "db_VNA"(w461) -> ()
        }
        frame "1" {
          n277 = local read "original Path"() -> (w465:path)
          n278 = Build Path(base path=w465, name or relative path="TXT" ("名称或相对路径")) -> (appended path=w464:path)
          n279 = Build Path(base path=w465, name or relative path="UpLoad1" ("名称或相对路径")) -> (appended path=w482:path)
          n280 = local read "db_VNA"() -> (w468:string)
          n281 = call <vilib>:"Check if File or Folder Exists.vi"("path"=w482) -> ("file or folder exists?"=w481:bool, "dup path"=w480:path)  [unwired: 8 in, 1 out]
          n282 = local read "S/N:"() -> (w479:string)
          n283 = List Folder(path=w464) -> (filenames=w474:string[])  [unwired: 3 in, 3 out]
          n284 = case shown="假" w481 {
            tunnel: w480 -> [w504 w505]
            tunnel: [w503 w505] -> w475
            frame False {
              n285 = Create Folder(path (use dialog)=w504) -> (created path=w503:path)  [unwired: 2 in, 2 out]
            }
            frame True {
            }
          }
          n286 = call <vilib>:"Trim Whitespace.vi"("string"=w479) -> ("trimmed string"=w478:string)  [unwired: 1 in]
          n287 = Concatenate Strings("P#", w478, "#Summary.zip") -> (w466:string)
          n288 = Concatenate Strings(w468, w466) -> (w467:string)
          n289 = Build Path(base path=w475, name or relative path=w466) -> (appended path=w473:path)
          n290 = local write "db_VNA"(w467) -> ()
          n291 = call <vilib>:"New Zip File.vi"("target"=w473) -> ("error out"=w470:errorcluster, "zip file out"=w472:i64)  [unwired: 4 in, 1 out]
          n292 = for {
            tunnel: w474 -> [w487] mode=indexing
            tunnel: w464 -> [w492]
            shift-right: [w490] -> w471
            shift-left: w472 -> [w491]
            shift-right: [w488] -> w469
            shift-left: w470 -> [w489]
            n293 = Search and Replace String(input string=w487, search string="Summary" ("搜索字符串")) -> (number of replacements=w486:i32)  [unwired: 6 in, 3 out]
            n294 = Greater Than 0?(x=w486) -> (x > 0?=w485:bool)
            n295 = case shown="真" w485 {
              tunnel: w492 -> [_ w502]
              tunnel: w491 -> [w494 w501]
              tunnel: [w494 w500] -> w490
              tunnel: w489 -> [w493 w497]
              tunnel: [w493 w496] -> w488
              tunnel: w487 -> [_ w495]
              frame False {
              }
              frame True {
                n296 = String To Path(string=w495) -> (path=w498:path)
                n297 = Build Path(base path=w502, name or relative path=w495) -> (appended path=w499:path)
                n298 = call <vilib>:"Add File to Zip.vi"("error in (no error)"=w497, "destination path in zip"=w498, "source file path"=w499, "zip file in"=w501) -> ("error out"=w496:errorcluster, "zip file out"=w500:i64)  [unwired: 6 in]
              }
            }
          }
          n299 = call <vilib>:"Close Zip File.vi"("error in (no error)"=w469, "zip file in"=w471) -> ()  [unwired: 5 in, 1 out]
        }
      }
    }
    frame #12 {
      # "生成txt的文件"
      n300 = flat-sequence {
        frame #0 {
          w509 = ";" ("搜索字符串/字符(-)")
          n301 = local read "db_VNA"() -> (w511:string)
          n302 = local read "条码输出"() -> (w508:string)
          n303 = Search/Split String(string=w511, search string/char (-)=w509) -> (substring before match=w510:string, match + rest of string=w506:string)  [unwired: 1 in, 1 out]
          n304 = Concatenate Strings(w510, w509, w508, w506) -> (w507:string)
          n305 = local write "db_VNA"(w507) -> ()
        }
        frame #1 {
          w513 = ";" ("搜索字符串/字符(-)")
          n306 = local read "db_VNA"() -> (w525:string)
          n307 = Concatenate Strings(w525, w513, "mis原始sn字符串", w513, "eprm_datecode", w513, "eprm_dateAndsn", w513, "itsn_really", w513, "label_date", w513, "label_sn", w513, "decimel_date", w513, "decimel_sn", w513, "MO", w513, "重测原因", w513, "测试模式", w513, "测试线别") -> (w526:string)
          n308 = local write "db_VNA"(w526) -> ()
        }
        frame #2 {
          n309 = local read "original Path"() -> (w530:path)
          n310 = Build Path(base path=w530, name or relative path="UpLoad1" ("名称或相对路径")) -> (appended path=w538:path)
          n311 = local read "S/N:"() -> (w535:string)
          n312 = call <vilib>:"Check if File or Folder Exists.vi"("path"=w538) -> ("file or folder exists?"=w537:bool, "dup path"=w536:path)  [unwired: 8 in, 1 out]
          n313 = call <vilib>:"Trim Whitespace.vi"("string"=w535) -> ("trimmed string"=w534:string)  [unwired: 1 in]
          n314 = case shown="真" w537 {
            tunnel: w536 -> [w541 w542]
            tunnel: [w540 w542] -> w531
            frame False {
              n315 = Create Folder(path (use dialog)=w541) -> (created path=w540:path)  [unwired: 2 in, 2 out]
            }
            frame True {
            }
          }
          n316 = Concatenate Strings("P#", w534, "#v.txt") -> (w529:string)
          n317 = local read "db_VNA"() -> (w527:string)
          n318 = Build Path(base path=w531, name or relative path=w529) -> (appended path=w528:path)
          n319 = Write to Text File(file (use dialog)=w528, text=w527) -> ()  [unwired: 2 in, 3 out]
        }
      }
    }
    frame #13 {
      n320 = flat-sequence {
        frame #0 {
          w550 = ";"
          n321 = local read "S/N:"() -> (w548:string)
          n322 = call <vilib>:"Trim Whitespace.vi"("string"=w548) -> ("trimmed string"=w547:string)  [unwired: 1 in]
          n323 = local read "original Path"() -> (w558:path)
          n324 = Concatenate Strings("P#", w547, "#s.zip") -> (w544:string)
          n325 = Build Path(base path=w558, name or relative path="UpLoad2" ("名称或相对路径")) -> (appended path=w566:path)
          n326 = call <vilib>:"Check if File or Folder Exists.vi"("path"=w566) -> ("file or folder exists?"=w565:bool, "dup path"=w564:path)  [unwired: 8 in, 1 out]
          n327 = local read "S/N:"() -> (w563:string)
          n328 = local read "P/N:"() -> (w554:string)
          n329 = local read "S/N:"() -> (w553:string)
          n330 = Format Date/Time String(time format string (%c)="%H:%M:%S %Y/%m/%d") -> (date/time string=w551:string)  [unwired: 2 in]
          n331 = case shown="假" w565 {
            tunnel: w564 -> [w569 w570]
            tunnel: [w568 w570] -> w559
            frame False {
              n332 = Create Folder(path (use dialog)=w569) -> (created path=w568:path)  [unwired: 2 in, 2 out]
            }
            frame True {
            }
          }
          n333 = call <vilib>:"Trim Whitespace.vi"("string"=w563) -> ("trimmed string"=w562:string)  [unwired: 1 in]
          n334 = Concatenate Strings("P#", w562, "#s.txt") -> (w557:string)
          n335 = Build Path(base path=w559, name or relative path=w557) -> (appended path=w556:path)
          n336 = Concatenate Strings(w554, w550, w553, w550, "L037407", w550, w551, w550, "PASS", w550, w544) -> (w549:string)
          n337 = Write to Text File(file (use dialog)=w556, text=w549) -> ()  [unwired: 2 in, 3 out]
        }
        frame #1 {
          n338 = local read "S/N:"() -> (w573:string)
          n339 = local read "original Path"() -> (w577:path)
          n340 = call <vilib>:"Trim Whitespace.vi"("string"=w573) -> ("trimmed string"=w574:string)  [unwired: 1 in]
          n341 = Concatenate Strings("UpLoad2\\" ("名称或相对路径"), "P#", w574, "#s.zip") -> (w571:string)
          n342 = Build Path(base path=w577, name or relative path=w571) -> (appended path=w578:path)
          n343 = call <vilib>:"New Zip File.vi"("target"=w578) -> ("zip file out"=w579:i64)  [unwired: 4 in, 2 out]
          n344 = call <vilib>:"Close Zip File.vi"("zip file in"=w579) -> ()  [unwired: 6 in, 1 out]
        }
      }
    }
    frame #14 {
      n345 = stacked-sequence {
        frame #0 {
          n346 = First Call?() -> (First Call?: T/F=w580:bool)
          n347 = case shown="真" w580 {
            frame False {
            }
            frame True {
              (unwired) "net use \\\\172.20.20.113 mesuser /user:mesuser" ("standard input")
              n348 = call <vilib>:"System Exec.vi"("command line"="NetCmdCompress") -> ()  [unwired: 7 in, 4 out]
            }
          }
        }
        frame #1 {
          (unwired) path "\\\\172.20.20.113\\emc/HPTS/VNA" ("目标路径（使用对话框）")
          n349 = local read "original Path"() -> (w586:path)
          n350 = Build Path(base path=w586, name or relative path="UpLoad1" ("名称或相对路径")) -> (appended path=w585:path)
          n351 = List Folder(path=w585) -> (path out=w583:path, filenames=w584:string[])  [unwired: 3 in, 2 out]
          n352 = for {
            tunnel: w584 -> [w590] mode=indexing
            tunnel: w583 -> [w591]
            tunnel: "NetPathCompress1" -> [w588]
            n353 = Build Path(base path=w591, name or relative path=w590) -> (appended path=w589:path)
            n354 = Copy(10:w588, 11:w589) -> ()  [unwired: 3 in, 3 out]
          }
        }
        frame #2 {
          (unwired) path "\\\\172.20.20.113\\emc/HPTS/SI" ("目标路径（使用对话框）")
          n355 = local read "original Path"() -> (w596:path)
          n356 = Build Path(base path=w596, name or relative path="UpLoad2" ("名称或相对路径")) -> (appended path=w595:path)
          n357 = List Folder(path=w595) -> (path out=w593:path, filenames=w594:string[])  [unwired: 3 in, 2 out]
          n358 = for {
            tunnel: w594 -> [w600] mode=indexing
            tunnel: w593 -> [w601]
            tunnel: "NetPathCompress2" -> [w598]
            n359 = Build Path(base path=w601, name or relative path=w600) -> (appended path=w599:path)
            n360 = Copy(10:w598, 11:w599) -> ()  [unwired: 3 in, 3 out]
          }
        }
      }
    }
  }
